vi "AddControl(s)ToControlStateArray.vi"   [LabVIEW 2017]
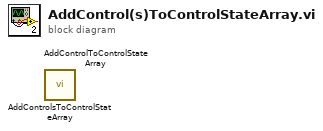
[diagram p0: block diagram]
diagram:
  n1 = call "AddControlsToControlStateArray.vi"() -> ()  [unwired: 10 in, 2 out]
  n2 = call "AddControlToControlStateArray.vi"() -> ()  [unwired: 10 in, 2 out]
